vi "draw_line_plot_imagesMOD.vi"() -> ()   [LabVIEW 2019]
uses:
  <vilib>/Analysis/NI_AALBase.lvlib
panel:
  in  "stop":bool
  out "XY Graph":cluster{i32[], "Sinusoidal Pattern":dbl[]}(graph)={[0, 1, 2, 3, 4, 5, 6, 7, 8, 9, 10, 11, 12, 13, 14, 15, 16, 17, 18, 19, 20, 21, 22, 23, 24, 25, 26, 27, 28, 29, 30, 31, 32, 33, 34, 35, 36, 37, 38, 39, 40, 41, 42, 43, 44, 45, 46, 47, 48, 49, 50, 51, 52, 53, 54, 55, 56, 57, 58, 59, 60, 61, 62, 63, 64, 65, 66, 67, 68, 69, 70, 71, 72, 73, 74, 75, 76, 77, 78, 79, 80, 81, 82, 83, 84, 85, 86, 87, 88, 89, 90, 91, 92, 93, 94, 95, 96, 97, 98, 99, 100, 101, 102, 103, 104, 105, 106, 107, 108, 109, 110, 111, 112, 113, 114, 115, 116, 117, 118, 119, 120, 121, 122, 123, 124, 125, 126, 127], "Sinusoidal Pattern"=[10.0, 10.049067674327418, 10.09801714032956, 10.146730474455362, 10.195090322016128, 10.242980179903263, 10.290284677254462, 10.33688985339222, 10.38268343236509, 10.427555093430282, 10.471396736825998, 10.514102744193222, 10.555570233019601, 10.595699304492433, 10.634393284163645, 10.671558954847018, 10.707106781186548, 10.74095112535496, 10.773010453362737, 10.803207531480645, 10.831469612302545, 10.857728610000272, 10.881921264348355, 10.903989293123443, 10.923879532511286, 10.94154406518302, 10.95694033573221, 10.970031253194545, 10.98078528040323, 10.989176509964782, 10.995184726672196, 10.998795456205173, 11.0, 10.998795456205173, 10.995184726672196, 10.989176509964782, 10.98078528040323, 10.970031253194545, 10.95694033573221, 10.94154406518302, 10.923879532511286, 10.903989293123443, 10.881921264348355, 10.857728610000272, 10.831469612302545, 10.803207531480645, 10.773010453362737, 10.74095112535496, 10.707106781186548, 10.671558954847018, 10.634393284163647, 10.595699304492435, 10.555570233019603, 10.514102744193222, 10.471396736825998, 10.427555093430282, 10.38268343236509, 10.33688985339222, 10.290284677254462, 10.242980179903265, 10.195090322016128, 10.146730474455362, 10.098017140329562, 10.049067674327418, 10.0, 9.950932325672582, 9.90198285967044, 9.853269525544638, 9.804909677983872, 9.757019820096737, 9.709715322745538, 9.66311014660778, 9.61731656763491, 9.572444906569718, 9.528603263174002, 9.485897255806778, 9.444429766980399, 9.404300695507567, 9.365606715836355, 9.328441045152982, 9.292893218813452, 9.25904887464504, 9.226989546637263, 9.196792468519355, 9.168530387697455, 9.142271389999728, 9.118078735651645, 9.096010706876557, 9.076120467488714, 9.05845593481698, 9.04305966426779, 9.029968746805455, 9.01921471959677, 9.010823490035218, 9.004815273327804, 9.001204543794827, 9.0, 9.001204543794827, 9.004815273327804, 9.010823490035218, 9.01921471959677, 9.029968746805455, 9.04305966426779, 9.058455934816978, 9.076120467488714, 9.096010706876555, 9.118078735651645, 9.142271389999728, 9.168530387697455, 9.196792468519355, 9.226989546637263, 9.25904887464504, 9.292893218813452, 9.328441045152982, 9.365606715836353, 9.404300695507565, 9.444429766980397, 9.485897255806778, 9.528603263174002, 9.572444906569718, 9.61731656763491, 9.66311014660778, 9.709715322745538, 9.757019820096735, 9.804909677983872, 9.853269525544638, 9.901982859670438, 9.950932325672582]}
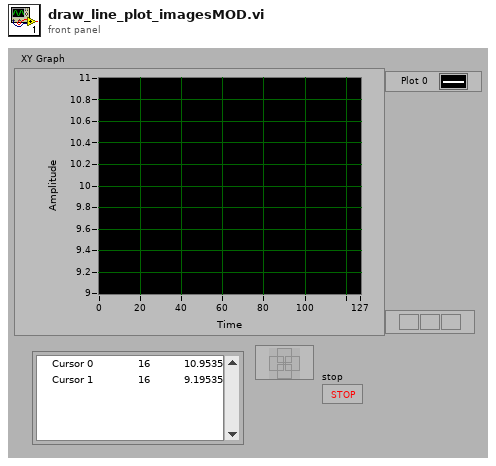
[diagram p1: front panel]
types:
  T1 = cluster{"Width":u16, "Style":enum32{"Solid", "Dash", "Dot", "DashDot", "DashDotDot"}}
  T2 = typedef "LVCursorListTypeDef.ctl" = cluster{"Name":string, "Color":u32, "Style":u8, "Point Style":u8, "Name Visible":bool, "Allow Drag":bool, "Cursor Mode":u32, "Plot":i32, "Index":i32, "Position":cluster{"X":dbl, "Y":dbl}, "X Scale":u32, "Y Scale":u32, "Watch Plots":i32[], "Watch All Plots":bool, "Plot Area":i32, "Label Offset":cluster{"X":dbl, "Y":dbl}}[]
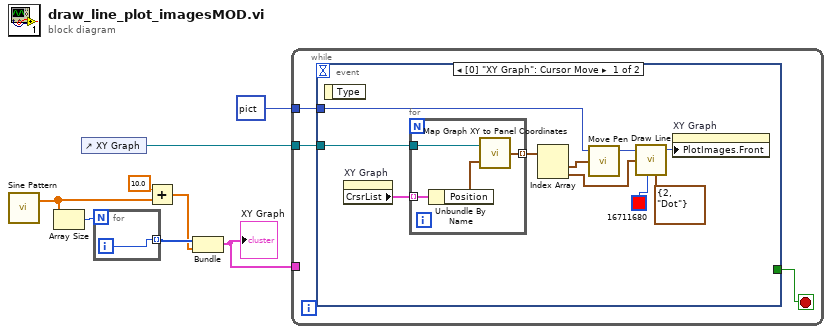
[diagram p0: block diagram]
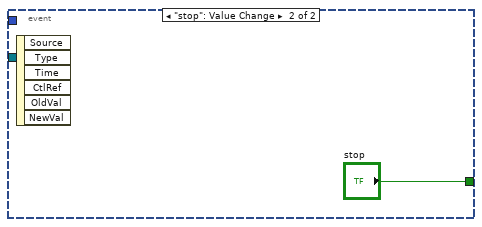
[diagram p2: hidden frame]
diagram:
  n1 = call <vilib>:"Sine Pattern.vi"() -> ("Sinusoidal Pattern"=w8:dbl[])  [unwired: 4 in, 1 out]
  n2 = Array Size(array=w8) -> (size(s)=w6:i32)
  n3 = control-ref of="XY Graph"() -> (w3:refnum<vi>)
  n4 = for {
    N: w6 -> [_]
    tunnel: [w9] -> w7 mode=indexing
    i -> [w9]
  }
  n5 = Add(x=10.0, y=w8) -> (x+y=w5:dbl[])
  n6 = Bundle(w7, w5) -> (w2:cluster{i32[], dbl[]})  [unwired: 1 in]
  "XY Graph" <- w2
  n7 = while {
    tunnel: w3 -> [w12]
    tunnel: w2 -> [_]
    tunnel: picture data[5B] ("picture") -> [w10]
    stop <- w11 stop-if-true
    n8 = event shown="[0] \"XY Graph\": Cursor Move" {
      selector: _ -> [_ _]
      dyn-events: _ -> [_ _]
      timeout: _ -> [_ _]
      tunnel: w12 -> [w16 _]
      tunnel: [_ "stop"] -> w11
      tunnel: w10 -> [w13 _]
      event "XY Graph": Cursor Move {
        n9 = event-data() -> ()  [unwired: 1 in, 1 out]
        n10 = property on="XY Graph" class="XYGraph (strict)"() -> ("CrsrList"=w22:T2)  [unwired: 2 in, 2 out]
        n11 = for {
          tunnel: w22 -> [w26] mode=indexing
          tunnel: [w24] -> w21 mode=indexing
          tunnel: w16 -> [w23]
          n12 = Unbundle By Name(w26) -> ("Position"=w25:cluster{"X":dbl, "Y":dbl})
          n13 = call "Map Graph XY to Panel Coordinates.vi"("XY"=w25, "Graph"=w23) -> ("Coords"=w24:cluster{i32, i32})
        }
        n14 = Index Array(array=w21) -> (element #1=w14:cluster{i32, i32}, element #2=w15:cluster{i32, i32})  [unwired: 2 in]
        n15 = call <vilib>:"Move Pen.vi"("new position"=w14, "picture"=w13) -> ("new picture"=w20:picture)  [unwired: 3 in]
        n16 = call <vilib>:"Draw Line.vi"("picture"=w20, "end point"=w15, "color(black)"=u32 16711680, "pen"=T1 {"Width"=2, "Style"=enum."Dot"}) -> ("new picture"=w19:picture)  [unwired: 5 in]
        n17 = property on="XY Graph" class="XYGraph (strict)"("PlotImages.Front"=w19) -> ()  [unwired: 2 in, 2 out]
      }
      event "stop": Value Change {
        n18 = event-data() -> ()  [unwired: 1 in, 6 out]
      }
    }
  }
